vi "Main_flow_full_clean.vi"() -> ()   [LabVIEW 2022 SP3]
uses:
  <vilib>/DAQmx/write.llb/DAQmx Write (Digital Bool 1Line 1Point).vi
  <vilib>/DAQmx/read.llb/DAQmx Read (Digital Bool 1Line 1Point).vi
  <vilib>/DAQmx/read.llb/DAQmx Read (Analog 1D DBL NChan 1Samp).vi
  <vilib>/DAQmx/create/channels.llb/DAQmx Create Channel (AI-Voltage-Basic).vi
  <vilib>/DAQmx/create/channels.llb/DAQmx Create Channel (DO-Digital Output).vi
  <vilib>/DAQmx/create/channels.llb/DAQmx Create Channel (DI-Digital Input).vi
  <vilib>/DAQmx/miscellaneous.llb/DAQmx Fill In Error Info.vi
panel:
  out "main loop executed":dbl
  out "Servo Angle":dbl(slide) scale=0.0..150.0
  in  "stop (F)":bool
  out "Square":dynamicdata(graph)
  in  "Frequency":dbl=50.0
  in  "Offset":dbl=2.5
  in  "Amplitude":dbl=2.5
  out "LDR Value":dbl
  in  "Relay 2":tag
  in  "Relay 1":tag
  out "Numeric 2":dbl
  out "Numeric":dbl
  in  "UP DOWN 2":tag
  in  "UP DOWN 1":tag
  in  "Buzzer":tag
  out "Counter":dbl
  out "OUT COUNT":dbl
  out "IN COUNT":dbl
  in  "Door IR 1 & 2 & LDR":tag
  in  "Trigger Period(sec)":dbl
  out "Current Time":dbl
  in  "Mode":dbl
  in  "stop":bool
  # "Dev1/ai4:6"
  # "Dev1/port0/line2"
  # "Dev1/port0/line0"
  # "Dev1/port0/line1"
  # "Dev1/port0/line3"
  # "Dev1/port0/line3"
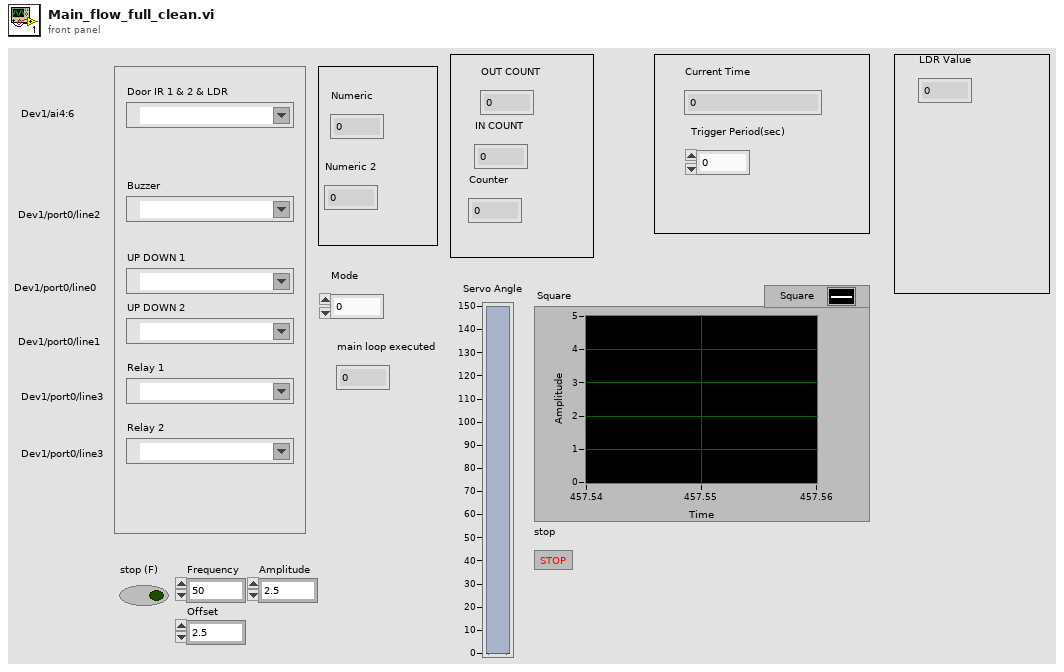
[diagram p1: front panel]
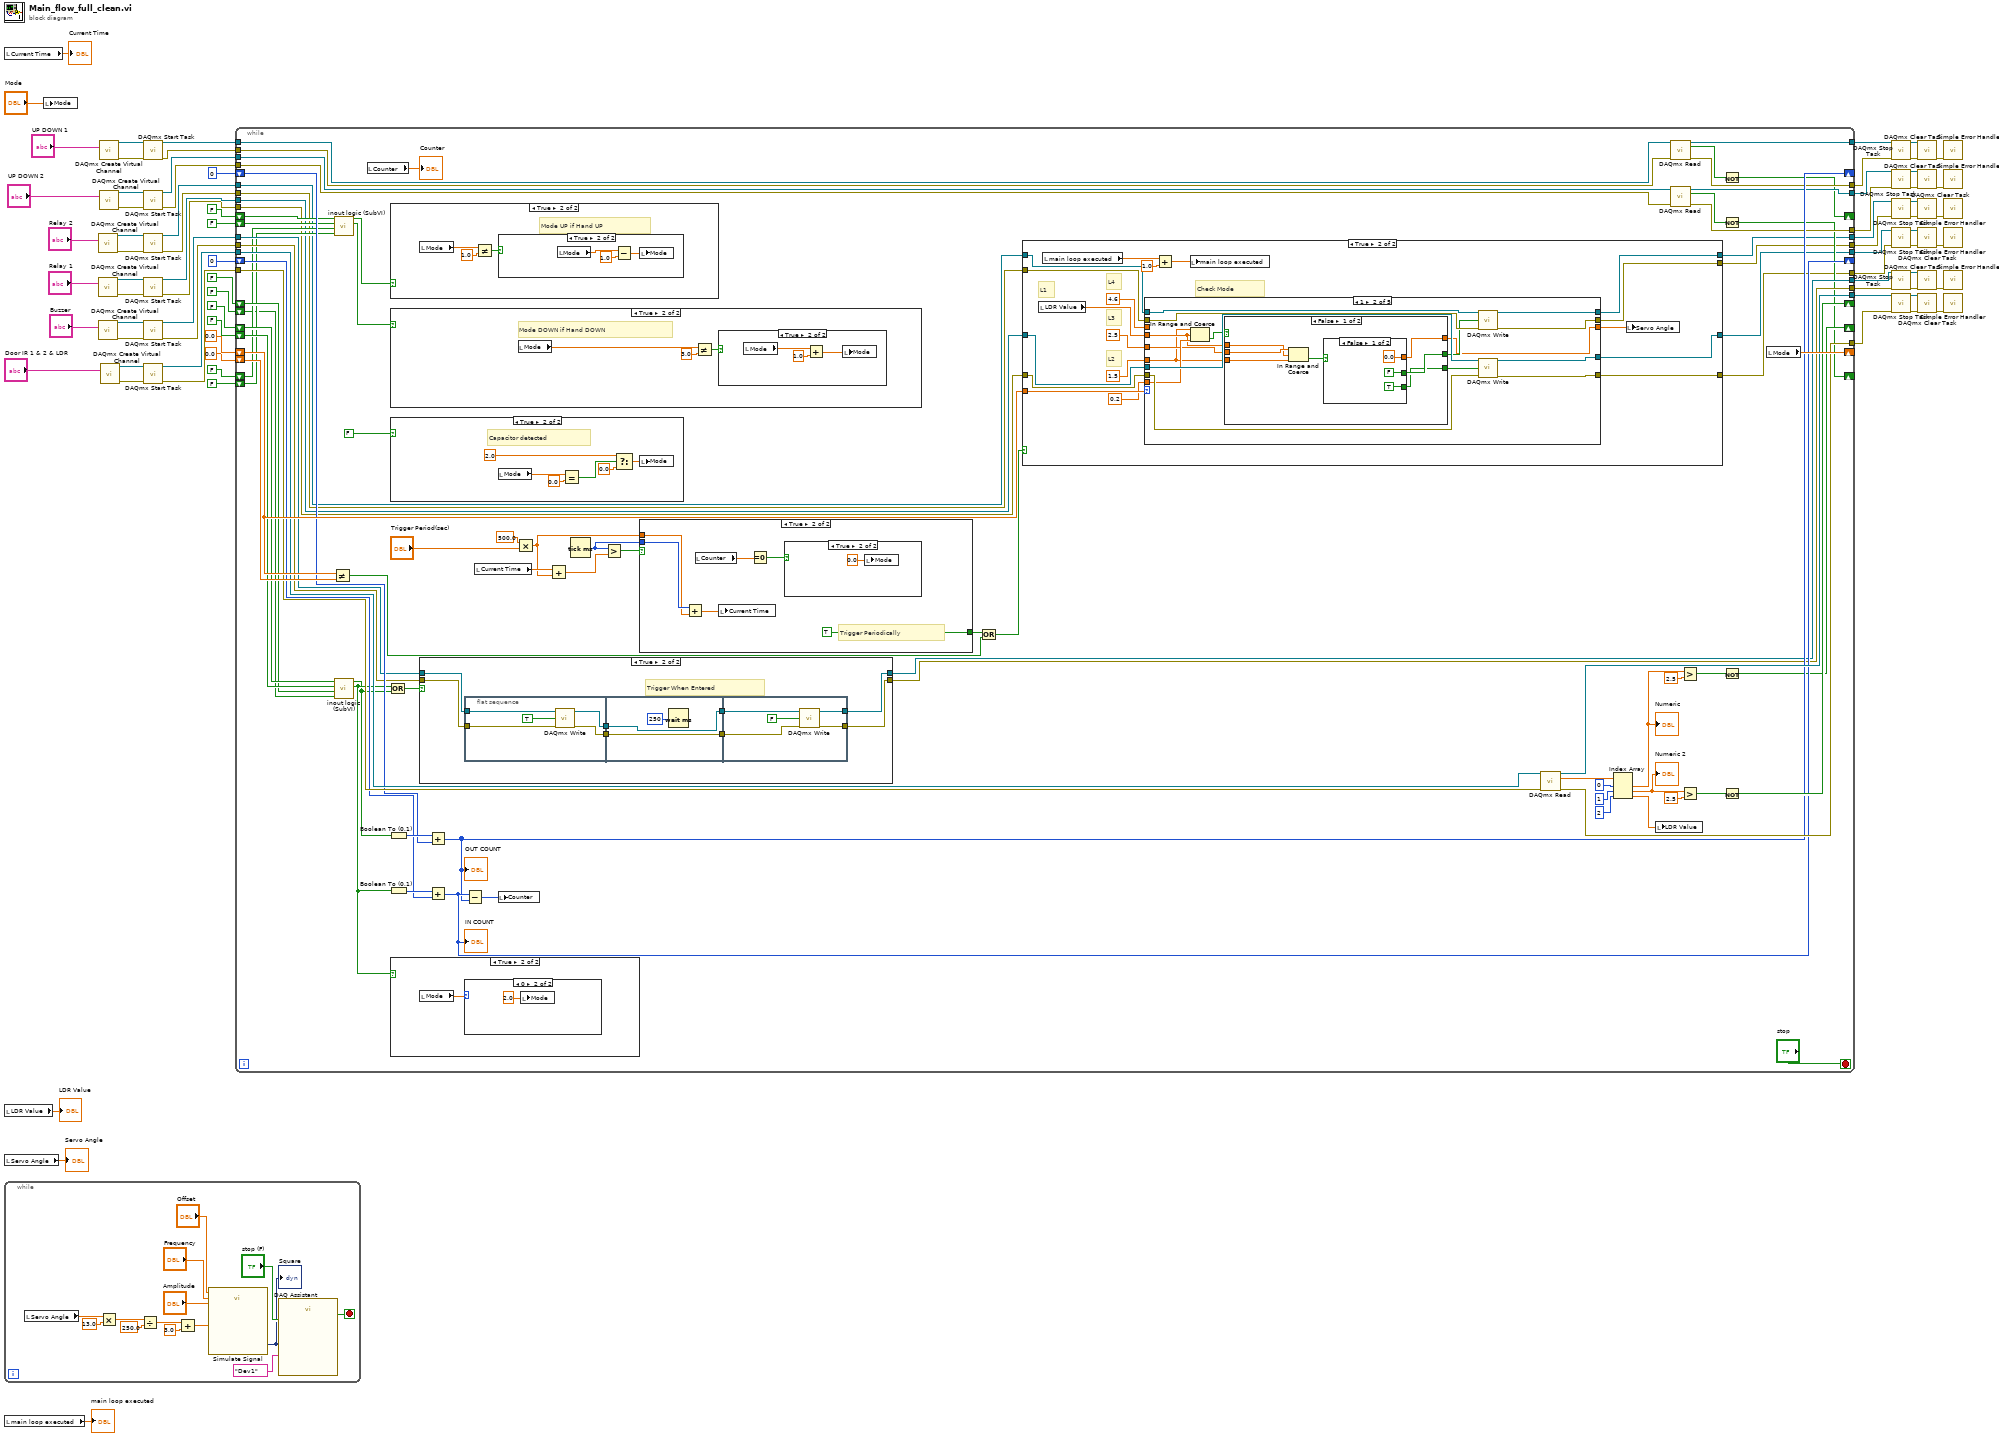
[diagram p0: block diagram]
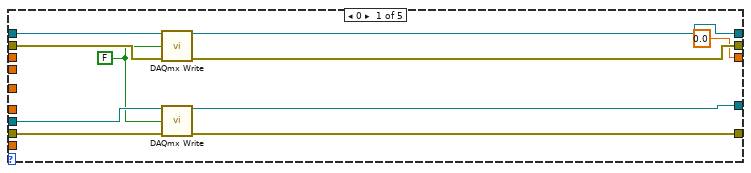
[diagram p5: hidden frame]
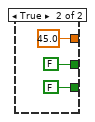
[diagram p6: hidden frame]
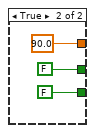
[diagram p7: hidden frame]
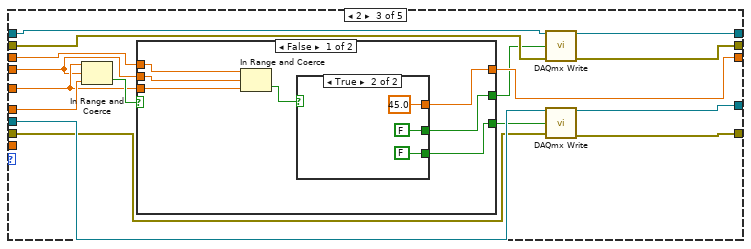
[diagram p8: hidden frame]
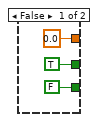
[diagram p9: hidden frame]
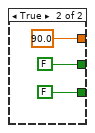
[diagram p10: hidden frame]
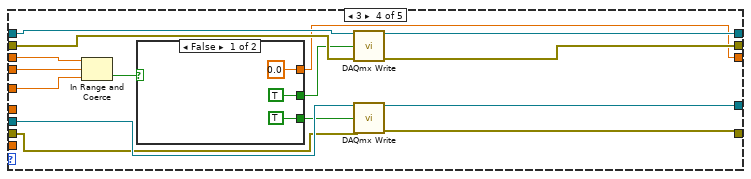
[diagram p11: hidden frame]
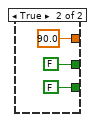
[diagram p12: hidden frame]
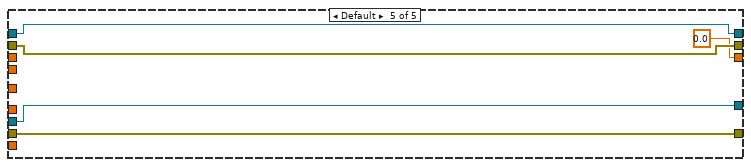
[diagram p13: hidden frame]
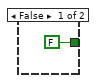
[diagram p18: hidden frame]
diagram:
  n1 = local read "Current Time"() -> (→"Current Time":dbl)
  n2 = local read "LDR Value"() -> (→"LDR Value":dbl)
  n3 = local read "Servo Angle"() -> (→"Servo Angle":dbl)
  n4 = while {
    stop <- w90 stop-if-true
    n5 = local read "Servo Angle"() -> (w78:dbl)
    n6 = Multiply(x=w78, y=13.0) -> (x*y=w84:dbl)
    n7 = Divide(x=w84, y=250.0) -> (x/y=w83:dbl)
    n8 = Add(x=w83, y=3.0) -> (x+y=w79:dbl)
    n9 = call "Simulate Signal"("Offset"="Offset", "Duty Cycle (%)"=w79, "Frequency"="Frequency", "Amplitude"="Amplitude") -> ("Square"=w86:dynamicdata)  [unwired: 10 in, 1 out]
    "Square" <- w86
    n10 = call "DAQ Assistant"("data"=w86, "stop (F)"="stop (F)", "device name"=tag "Dev1") -> ("stopped"=w90:bool)  [unwired: 14 in, 2 out]
  }
  n11 = local read "main loop executed"() -> (→"main loop executed":dbl)
  n12 = local write "Mode"("Mode") -> ()
  n13 = call-poly <vilib>:"DAQmx Create Virtual Channel.vi"("lines"="Relay 2") -> ("task out"=w19:refnum<k21>, "error out"=w18:errorcluster)  [unwired: 13 in]
  n14 = call-poly <vilib>:"DAQmx Create Virtual Channel.vi"("lines"="Relay 1") -> ("task out"=w22:refnum<k21>, "error out"=w21:errorcluster)  [unwired: 13 in]
  n15 = call-poly <vilib>:"DAQmx Create Virtual Channel.vi"("lines"="Buzzer") -> ("task out"=w58:refnum<k21>, "error out"=w56:errorcluster)  [unwired: 13 in]
  n16 = call-poly <vilib>:"DAQmx Create Virtual Channel.vi"("lines"="UP DOWN 1") -> ("task out"=w48:refnum<k21>, "error out"=w46:errorcluster)  [unwired: 13 in]
  n17 = call-poly <vilib>:"DAQmx Create Virtual Channel.vi"("lines"="UP DOWN 2") -> ("task out"=w47:refnum<k21>, "error out"=w45:errorcluster)  [unwired: 13 in]
  n18 = call-poly <vilib>:"DAQmx Create Virtual Channel.vi"("physical channels"="Door IR 1 & 2 & LDR") -> ("task out"=w73:refnum<k21>, "error out"=w70:errorcluster)  [unwired: 13 in]
  n19 = call <vilib>:"DAQmx Start Task.vi"("task/channels in"=w48, "error in"=w46) -> ("task out"=w42:refnum<k21>, "error out"=w41:errorcluster)  [unwired: 12 in]
  n20 = call <vilib>:"DAQmx Start Task.vi"("task/channels in"=w47, "error in"=w45) -> ("task out"=w40:refnum<k21>, "error out"=w39:errorcluster)  [unwired: 12 in]
  n21 = call <vilib>:"DAQmx Start Task.vi"("task/channels in"=w19, "error in"=w18) -> ("task out"=w14:refnum<k21>, "error out"=w13:errorcluster)  [unwired: 12 in]
  n22 = call <vilib>:"DAQmx Start Task.vi"("task/channels in"=w22, "error in"=w21) -> ("task out"=w16:refnum<k21>, "error out"=w15:errorcluster)  [unwired: 12 in]
  n23 = call <vilib>:"DAQmx Start Task.vi"("task/channels in"=w58, "error in"=w56) -> ("task out"=w55:refnum<k21>, "error out"=w54:errorcluster)  [unwired: 12 in]
  n24 = call <vilib>:"DAQmx Start Task.vi"("task/channels in"=w73, "error in"=w70) -> ("task out"=w71:refnum<k21>, "error out"=w69:errorcluster)  [unwired: 12 in]
  n25 = while {
    shift-right: [w160] -> _
    shift-left: 0.0 ("Mode") -> [w158]
    shift-left: 0.0 ("Mode") -> [w159]
    tunnel: w71 -> [w155]
    tunnel: w69 -> [w154]
    tunnel: [w153] -> w68
    tunnel: [w152] -> w67
    shift-right: [w143] -> _
    shift-left: FALSE -> [w151]
    shift-left: FALSE -> [w150]
    shift-right: [w146] -> _
    shift-left: FALSE -> [w149]
    shift-left: FALSE -> [w120]
    shift-right: [w145] -> _
    shift-left: 0 -> [w148]
    shift-right: [w144] -> _
    shift-left: 0 -> [w147]
    tunnel: w55 -> [w140]
    tunnel: w54 -> [w139]
    tunnel: [w138] -> w50
    tunnel: [w137] -> w49
    shift-right: [w126] -> _
    shift-left: FALSE -> [w124]
    shift-right: [w125] -> _
    shift-left: FALSE -> [w122]
    shift-left: FALSE -> [w123]
    shift-left: FALSE -> [w121]
    tunnel: w42 -> [w134]
    tunnel: w41 -> [w133]
    tunnel: w40 -> [w132]
    tunnel: w39 -> [w131]
    tunnel: [w130] -> w32
    tunnel: [w129] -> w31
    tunnel: [w128] -> w30
    tunnel: [w127] -> w29
    tunnel: w16 -> [w102]
    tunnel: w15 -> [w101]
    tunnel: w14 -> [w100]
    tunnel: w13 -> [w99]
    tunnel: [w98] -> w6
    tunnel: [w97] -> w5
    tunnel: [w96] -> w4
    tunnel: [w95] -> w3
    stop <- "stop" stop-if-true
    n26 = Not Equal?(x=w158, y=w159) -> (x != y?=w94:bool)
    n27 = call "inout logic (SubVI).vi"("Sensor 2 (T-2)"=w121, "Sensor 2 (T-1)"=w122, "Sensor 1 (T-2)"=w123, "Sensor 1 (T-1)"=w124) -> ("IN"=w119:bool, "OUT"=w118:bool)  [unwired: 6 in]
    n28 = call "inout logic (SubVI).vi"("Sensor 2 (T-2)"=w120, "Sensor 2 (T-1)"=w149, "Sensor 1 (T-2)"=w150, "Sensor 1 (T-1)"=w151) -> ("IN"=w107:bool, "OUT"=w106:bool)  [unwired: 6 in]
    n29 = local read "Counter"() -> (→"Counter":dbl)
    n30 = Or(x=w107, y=w106) -> (x .or. y?=w105:bool)
    n31 = Boolean To (0,1)(Boolean=w106) -> (0, 1=w156:i16)
    n32 = Boolean To (0,1)(Boolean=w107) -> (0, 1=w157:i16)
    n33 = case shown="True" w118 {
      frame False {
      }
      frame True {
        # "Mode UP if Hand UP"
        n34 = local read "Mode"() -> (w295:dbl)
        n35 = Not Equal?(x=w295, y=1.0) -> (x != y?=w294:bool)
        n36 = case shown="True" w294 {
          frame False {
          }
          frame True {
            n37 = local read "Mode"() -> (w297:dbl)
            n38 = Subtract(x=w297, y=1.0) -> (x-y=w296:dbl)
            n39 = local write "Mode"(w296) -> ()
          }
        }
      }
    }
    n40 = case shown="True" w119 {
      frame False {
      }
      frame True {
        # "Mode DOWN if Hand DOWN"
        n41 = local read "Mode"() -> (w301:dbl)
        n42 = Not Equal?(x=w301, y=3.0) -> (x != y?=w299:bool)
        n43 = case shown="True" w299 {
          frame False {
          }
          frame True {
            n44 = local read "Mode"() -> (w304:dbl)
            n45 = Add(x=w304, y=1.0) -> (x+y=w302:dbl)
            n46 = local write "Mode"(w302) -> ()
          }
        }
      }
    }
    n47 = case shown="True" FALSE {
      frame False {
      }
      frame True {
        # "Capacitor detected"
        n48 = local read "Mode"() -> (w341:dbl)
        n49 = Equal?(x=w341, y=0.0) -> (x = y?=w339:bool)
        n50 = Select(t=2.0, s=w339, f=0.0) -> (s? t:f=w338:dbl)
        n51 = local write "Mode"(w338) -> ()
      }
    }
    n52 = case shown="True" w107 {
      frame False {
      }
      frame True {
        n53 = local read "Mode"() -> (w169:dbl)
        n54 = case shown="0" w169 {
          frame Default {
          }
          frame 0 {
            n55 = local write "Mode"(2.0 ("Mode")) -> ()
          }
        }
      }
    }
    n56 = case shown="True" w105 {
      tunnel: w140 -> [w313 w322]
      tunnel: w139 -> [w314 w321]
      tunnel: [w313 w316] -> w138
      tunnel: [w314 w315] -> w137
      frame False {
      }
      frame True {
        # "Trigger When Entered"
        n57 = flat-sequence {
          tunnel: w322 -> [w326]
          tunnel: w321 -> [w325]
          tunnel: [w324] -> w319
          tunnel: [w323] -> w317
          tunnel: [w329] -> w320
          tunnel: w319 -> [w329]
          tunnel: [w328] -> w318
          tunnel: w317 -> [w328]
          tunnel: w320 -> [w334]
          tunnel: w318 -> [w333]
          tunnel: [w332] -> w316
          tunnel: [w331] -> w315
          frame #0 {
            n58 = call-poly <vilib>:"DAQmx Write.vi"("task/channels in"=w326, "data"=TRUE, "error in"=w325) -> ("task out"=w324:refnum<k21>, "error out"=w323:errorcluster)  [unwired: 10 in, 1 out]
          }
          frame #1 {
            n59 = Wait (ms)(milliseconds to wait=u32 250) -> ()  [unwired: 1 out]
          }
          frame #2 {
            n60 = call-poly <vilib>:"DAQmx Write.vi"("task/channels in"=w334, "data"=FALSE, "error in"=w333) -> ("task out"=w332:refnum<k21>, "error out"=w331:errorcluster)  [unwired: 10 in, 1 out]
          }
        }
      }
    }
    n61 = Add(x=w156, y=w147) -> (x+y=w144:i32)
    "OUT COUNT" <- w144
    n62 = Add(x=w157, y=w148) -> (x+y=w145:i32)
    "IN COUNT" <- w145
    n63 = Subtract(x=w145, y=w144) -> (x-y=w142:i32)
    n64 = local read "Current Time"() -> (w167:dbl)
    n65 = local write "Counter"(w142) -> ()
    n66 = Multiply(x=500.0, y="Trigger Period(sec)") -> (x*y=w161:dbl)
    n67 = Add(x=w167, y=w161) -> (x+y=w164:dbl)
    n68 = Tick Count (ms)() -> (millisecond timer value=w165:u32)
    n69 = Greater?(x=w165, y=w164) -> (0:w166:bool)
    n70 = case shown="True" w166 {
      tunnel: w165 -> [_ w310]
      tunnel: w161 -> [_ w309]
      tunnel: [FALSE ("Check") TRUE ("Check")] -> w92
      frame False {
      }
      frame True {
        # "Trigger Periodically"
        n71 = Add(x=w310, y=w309) -> (x+y=w311:dbl)
        n72 = local read "Counter"() -> (w308:dbl)
        n73 = local write "Current Time"(w311) -> ()
        n74 = Equal To 0?(x=w308) -> (x = 0?=w307:bool)
        n75 = case shown="True" w307 {
          frame False {
          }
          frame True {
            n76 = local write "Mode"(0.0 ("Mode")) -> ()
          }
        }
      }
    }
    n77 = Or(x=w92, y=w94) -> (x .or. y?=w93:bool)
    n78 = case shown="True" w93 {
      tunnel: w158 -> [_ w192]
      tunnel: w102 -> [w174 w191]
      tunnel: w101 -> [w173 w190]
      tunnel: w100 -> [w172 w189]
      tunnel: w99 -> [w171 w188]
      tunnel: [w174 w187] -> w98
      tunnel: [w173 w186] -> w97
      tunnel: [w172 w185] -> w96
      tunnel: [w171 w184] -> w95
      frame False {
      }
      frame True {
        # "L4"
        # "L1"
        # "L3"
        # "L2"
        # "Check Mode"
        n79 = local read "LDR Value"() -> (w182:dbl)
        n80 = local read "main loop executed"() -> (w177:dbl)
        n81 = case shown="1" w192 {
          tunnel: w191 -> [w202 w218 w250 w281 w292]
          tunnel: w190 -> [w201 w216 w249 w280 w291]
          tunnel: w189 -> [w200 w214 w248 w279 w290]
          tunnel: w188 -> [w199 w212 w247 w278 w289]
          tunnel: [w198 w217 w246 w277 w292] -> w187
          tunnel: [w197 w215 w245 w276 w291] -> w186
          tunnel: [w196 w213 w244 w275 w290] -> w185
          tunnel: [w195 w211 w243 w274 w289] -> w184
          tunnel: 1.5 -> [_ w206 w242 _ _]
          tunnel: 0.2 -> [_ w209 _ _ _]
          tunnel: w182 -> [_ w207 w235 w270 _]
          tunnel: 2.5 -> [_ w208 w236 w271 _]
          tunnel: 4.6 -> [_ _ w237 w272 _]
          tunnel: [0.0 ("Servo Angle") w203 w240 w269 0.0 ("A")] -> w178
          frame 0 {
            w194 = FALSE ("data")
            n82 = call-poly <vilib>:"DAQmx Write.vi"("task/channels in"=w200, "data"=w194, "error in"=w199) -> ("task out"=w196:refnum<k21>, "error out"=w195:errorcluster)  [unwired: 10 in, 1 out]
            n83 = call-poly <vilib>:"DAQmx Write.vi"("task/channels in"=w202, "data"=w194, "error in"=w201) -> ("task out"=w198:refnum<k21>, "error out"=w197:errorcluster)  [unwired: 10 in, 1 out]
          }
          frame 1 {
            n84 = In Range and Coerce(upper limit=w206, x=w207, lower limit=w209) -> (In Range?=w210:bool)  [unwired: 1 out]
            n85 = case shown="False" w210 {
              tunnel: [w221 90.0] -> w203
              tunnel: [w220 FALSE] -> w204
              tunnel: [w219 FALSE] -> w205
              tunnel: w208 -> [w225 _]
              tunnel: w206 -> [w224 _]
              tunnel: w207 -> [w223 _]
              frame False {
                n86 = In Range and Coerce(upper limit=w225, x=w223, lower limit=w224) -> (In Range?=w222:bool)  [unwired: 1 out]
                n87 = case shown="False" w222 {
                  tunnel: [0.0 45.0] -> w221
                  tunnel: [FALSE FALSE] -> w220
                  tunnel: [TRUE FALSE] -> w219
                  frame False {
                  }
                  frame True {
                  }
                }
              }
              frame True {
              }
            }
            n88 = call-poly <vilib>:"DAQmx Write.vi"("task/channels in"=w214, "data"=w204, "error in"=w212) -> ("task out"=w213:refnum<k21>, "error out"=w211:errorcluster)  [unwired: 10 in, 1 out]
            n89 = call-poly <vilib>:"DAQmx Write.vi"("task/channels in"=w218, "data"=w205, "error in"=w216) -> ("task out"=w217:refnum<k21>, "error out"=w215:errorcluster)  [unwired: 10 in, 1 out]
          }
          frame 2 {
            n90 = In Range and Coerce(upper limit=w236, x=w235, lower limit=w242) -> (In Range?=w241:bool)  [unwired: 1 out]
            n91 = case shown="False" w241 {
              tunnel: [w253 90.0] -> w240
              tunnel: [w252 FALSE] -> w239
              tunnel: [w251 FALSE] -> w238
              tunnel: w237 -> [w257 _]
              tunnel: w236 -> [w256 _]
              tunnel: w235 -> [w255 _]
              frame False {
                n92 = In Range and Coerce(upper limit=w257, x=w255, lower limit=w256) -> (In Range?=w254:bool)  [unwired: 1 out]
                n93 = case shown="True" w254 {
                  tunnel: [0.0 45.0] -> w253
                  tunnel: [FALSE FALSE] -> w252
                  tunnel: [TRUE FALSE] -> w251
                  frame False {
                  }
                  frame True {
                  }
                }
              }
              frame True {
              }
            }
            n94 = call-poly <vilib>:"DAQmx Write.vi"("task/channels in"=w248, "data"=w238, "error in"=w247) -> ("task out"=w244:refnum<k21>, "error out"=w243:errorcluster)  [unwired: 10 in, 1 out]
            n95 = call-poly <vilib>:"DAQmx Write.vi"("task/channels in"=w250, "data"=w239, "error in"=w249) -> ("task out"=w246:refnum<k21>, "error out"=w245:errorcluster)  [unwired: 10 in, 1 out]
          }
          frame 3 {
            n96 = In Range and Coerce(upper limit=w272, x=w270, lower limit=w271) -> (In Range?=w273:bool)  [unwired: 1 out]
            n97 = case shown="False" w273 {
              tunnel: [0.0 90.0] -> w269
              tunnel: [TRUE FALSE] -> w268
              tunnel: [TRUE FALSE] -> w267
              frame False {
              }
              frame True {
              }
            }
            n98 = call-poly <vilib>:"DAQmx Write.vi"("task/channels in"=w279, "data"=w267, "error in"=w278) -> ("task out"=w275:refnum<k21>, "error out"=w274:errorcluster)  [unwired: 10 in, 1 out]
            n99 = call-poly <vilib>:"DAQmx Write.vi"("task/channels in"=w281, "data"=w268, "error in"=w280) -> ("task out"=w277:refnum<k21>, "error out"=w276:errorcluster)  [unwired: 10 in, 1 out]
          }
          frame Default {
          }
        }
        n100 = Add(x=w177, y=1.0) -> (x+y=w175:dbl)
        n101 = local write "main loop executed"(w175) -> ()
        n102 = local write "Servo Angle"(w178) -> ()
      }
    }
    n103 = call-poly <vilib>:"DAQmx Read.vi"("task/channels in"=w155, "error in"=w154) -> ("task out"=w153:refnum<k21>, "data"=w112:dbl[], "error out"=w152:errorcluster)  [unwired: 11 in]
    n104 = Index Array(array=w112, index #1=0 ("index"), index #2=1 ("index"), index #3=2 ("index")) -> (element #1=w111:dbl, element #2=w108:dbl, element #3=w103:dbl)
    "Numeric" <- w111
    "Numeric 2" <- w108
    n105 = local write "LDR Value"(w103) -> ()
    n106 = call-poly <vilib>:"DAQmx Read.vi"("task/channels in"=w134, "error in"=w133) -> ("task out"=w130:refnum<k21>, "data"=w136:bool, "error out"=w129:errorcluster)  [unwired: 11 in]
    n107 = call-poly <vilib>:"DAQmx Read.vi"("task/channels in"=w132, "error in"=w131) -> ("task out"=w128:refnum<k21>, "data"=w135:bool, "error out"=w127:errorcluster)  [unwired: 11 in]
    n108 = Greater?(x=w111, y=2.5) -> (0:w116:bool)
    n109 = Greater?(x=w108, y=2.5) -> (0:w114:bool)
    n110 = Not(x=w136) -> (.not. x?=w126:bool)
    n111 = Not(x=w135) -> (.not. x?=w125:bool)
    n112 = Not(x=w116) -> (.not. x?=w143:bool)
    n113 = Not(x=w114) -> (.not. x?=w146:bool)
    n114 = local read "Mode"() -> (w160:dbl)
  }
  n115 = call <vilib>:"DAQmx Stop Task.vi"("task/channels in"=w32, "error in"=w31) -> ("task out"=w38:refnum<k21>, "error out"=w36:errorcluster)  [unwired: 12 in]
  n116 = call <vilib>:"DAQmx Stop Task.vi"("task/channels in"=w30, "error in"=w29) -> ("task out"=w35:refnum<k21>, "error out"=w33:errorcluster)  [unwired: 12 in]
  n117 = call <vilib>:"DAQmx Stop Task.vi"("task/channels in"=w4, "error in"=w3) -> ("task out"=w9:refnum<k21>, "error out"=w7:errorcluster)  [unwired: 12 in]
  n118 = call <vilib>:"DAQmx Stop Task.vi"("task/channels in"=w6, "error in"=w5) -> ("task out"=w12:refnum<k21>, "error out"=w10:errorcluster)  [unwired: 12 in]
  n119 = call <vilib>:"DAQmx Stop Task.vi"("task/channels in"=w50, "error in"=w49) -> ("task out"=w53:refnum<k21>, "error out"=w51:errorcluster)  [unwired: 12 in]
  n120 = call <vilib>:"DAQmx Stop Task.vi"("task/channels in"=w68, "error in"=w67) -> ("task out"=w66:refnum<k21>, "error out"=w65:errorcluster)  [unwired: 12 in]
  n121 = call <vilib>:"DAQmx Clear Task.vi"("task in"=w38, "error in"=w36) -> ("error out"=w37:errorcluster)  [unwired: 13 in]
  n122 = call <vilib>:"DAQmx Clear Task.vi"("task in"=w35, "error in"=w33) -> ("error out"=w34:errorcluster)  [unwired: 13 in]
  n123 = call <vilib>:"DAQmx Clear Task.vi"("task in"=w9, "error in"=w7) -> ("error out"=w8:errorcluster)  [unwired: 13 in]
  n124 = call <vilib>:"DAQmx Clear Task.vi"("task in"=w12, "error in"=w10) -> ("error out"=w11:errorcluster)  [unwired: 13 in]
  n125 = call <vilib>:"DAQmx Clear Task.vi"("task in"=w53, "error in"=w51) -> ("error out"=w52:errorcluster)  [unwired: 13 in]
  n126 = call <vilib>:"DAQmx Clear Task.vi"("task in"=w66, "error in"=w65) -> ("error out"=w64:errorcluster)  [unwired: 13 in]
  n127 = call <vilib>:"Simple Error Handler.vi"("error in (no error)"=w37) -> ()  [unwired: 4 in, 5 out]
  n128 = call <vilib>:"Simple Error Handler.vi"("error in (no error)"=w34) -> ()  [unwired: 4 in, 5 out]
  n129 = call <vilib>:"Simple Error Handler.vi"("error in (no error)"=w8) -> ()  [unwired: 4 in, 5 out]
  n130 = call <vilib>:"Simple Error Handler.vi"("error in (no error)"=w11) -> ()  [unwired: 4 in, 5 out]
  n131 = call <vilib>:"Simple Error Handler.vi"("error in (no error)"=w52) -> ()  [unwired: 4 in, 5 out]
  n132 = call <vilib>:"Simple Error Handler.vi"("error in (no error)"=w64) -> ()  [unwired: 4 in, 5 out]
